vi "Receiver UI.vi"(8 "Error In":errorcluster) -> (0 "Error Out":errorcluster, 11 "Notification":bool)   [LabVIEW 2023, in "Receiver.lvclass"]
doc: "The VI receives data from sender and displays the received message of different data types."
uses:
  Receiver.lvclass
  Controls/Queue Operation.ctl
  Controls/User Event Operations.ctl
  Controls/Receiver Data.ctl
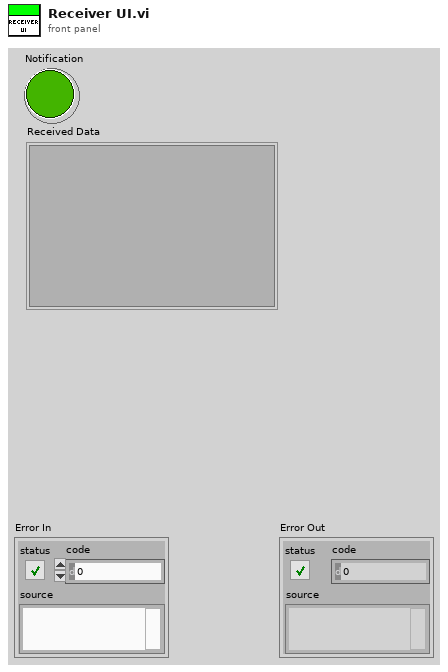
[diagram p1: front panel]
types:
  T1 = typedef "Receiver Data.ctl" = cluster{"Notification":bool, "Display Ref":refnum<vi>}
  T2 = typedef "User Event Operations.ctl" = enum16{"Obtain", "Generate", "Destroy"}
  T3 = typedef "Queue Operation.ctl" = enum16{"Create & Enqueue N", "Enqueue N", "Dequeue", "Enstack N", "Flush", "Release"}
  T4 = typedef "Queue Element.ctl" = cluster{"State":string, "Data":variant}
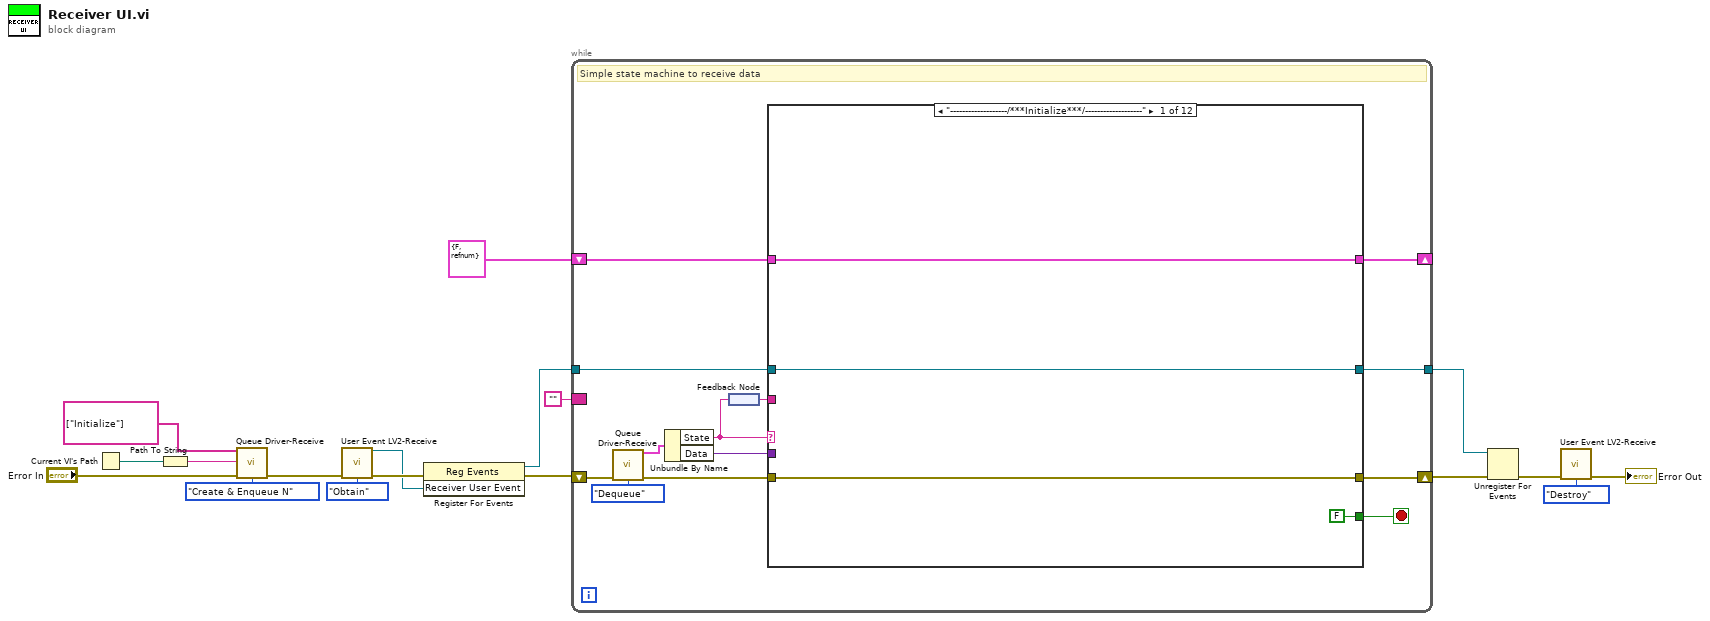
[diagram p0: block diagram]
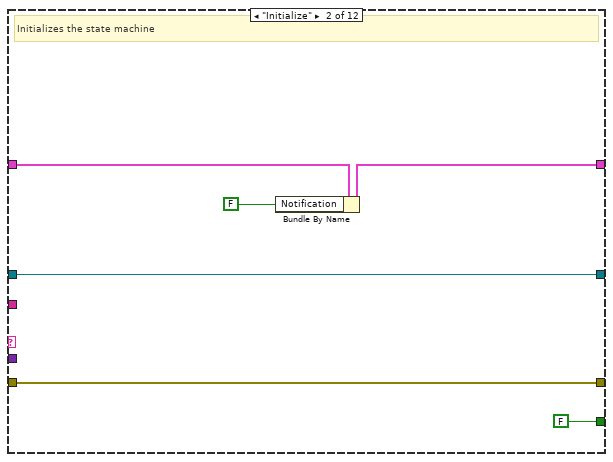
[diagram p2: hidden frame]
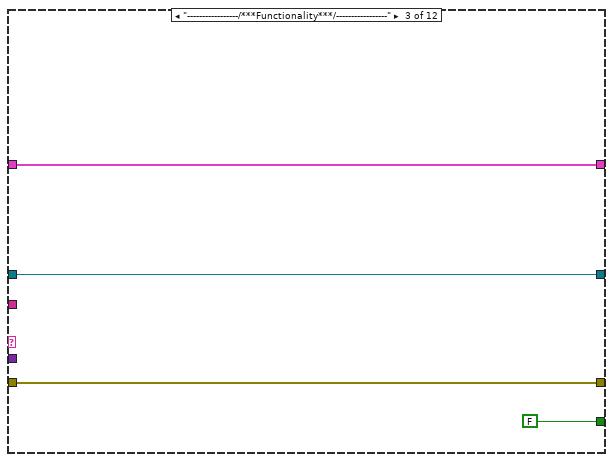
[diagram p3: hidden frame]
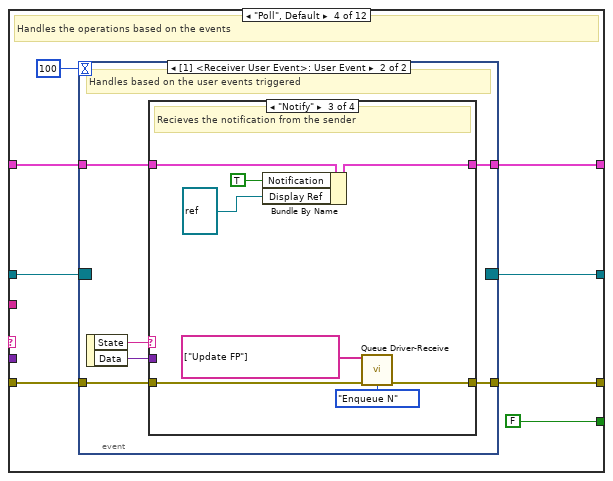
[diagram p4: hidden frame]
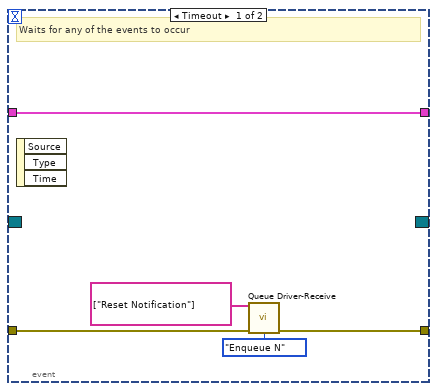
[diagram p5: hidden frame]
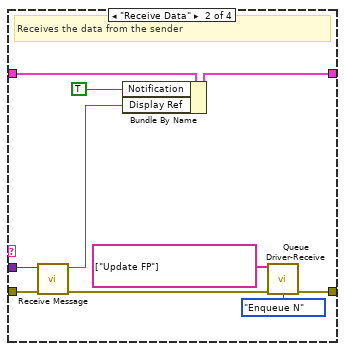
[diagram p7: hidden frame]
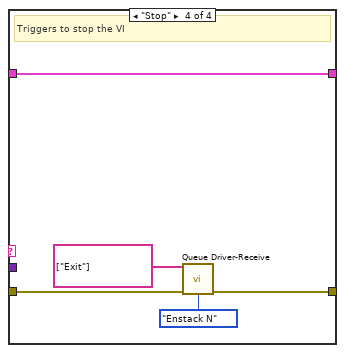
[diagram p8: hidden frame]
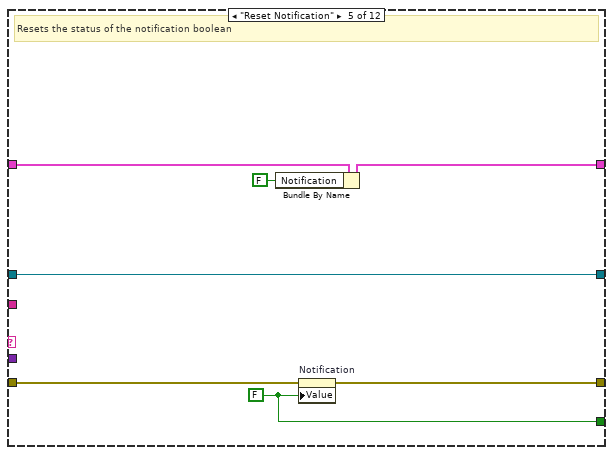
[diagram p9: hidden frame]
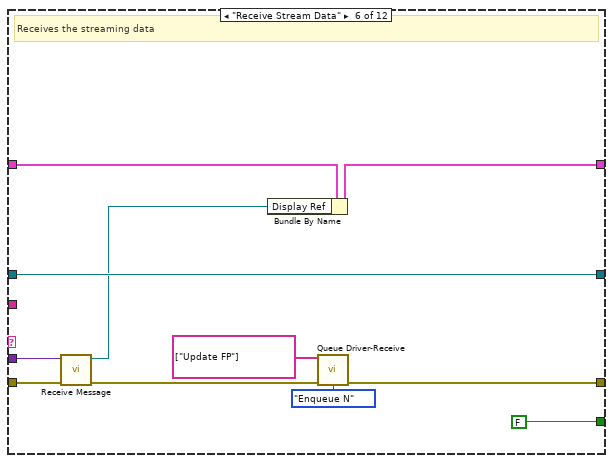
[diagram p10: hidden frame]
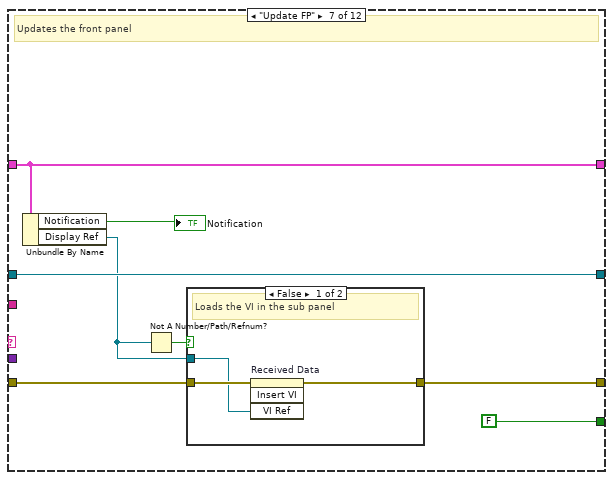
[diagram p11: hidden frame]
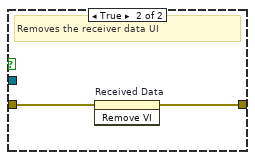
[diagram p12: hidden frame]
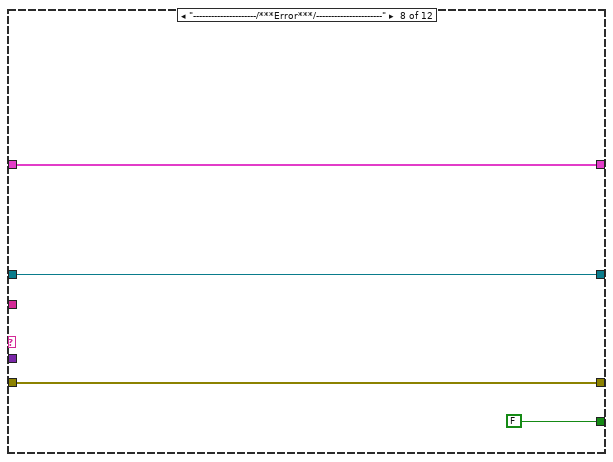
[diagram p13: hidden frame]
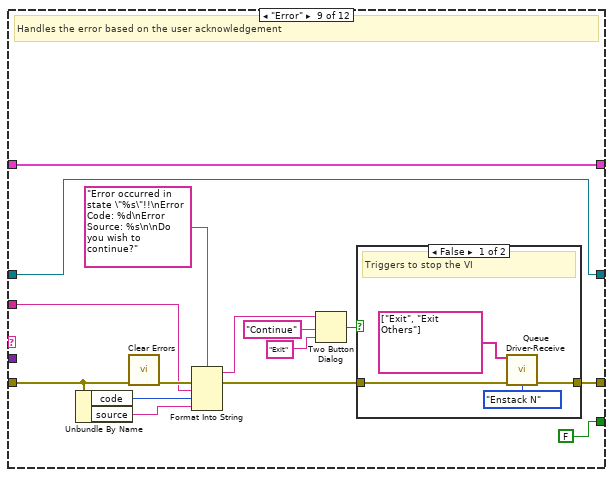
[diagram p14: hidden frame]
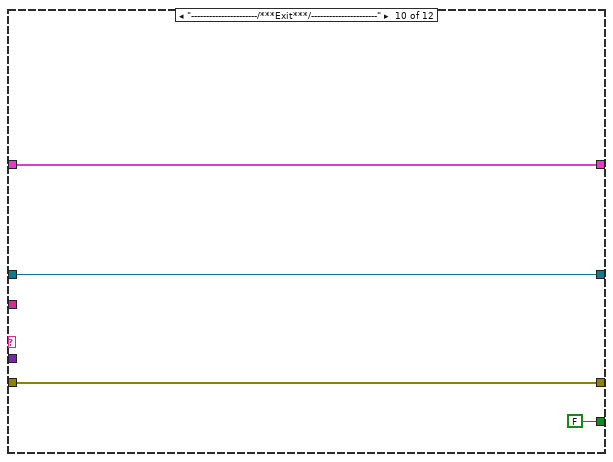
[diagram p16: hidden frame]
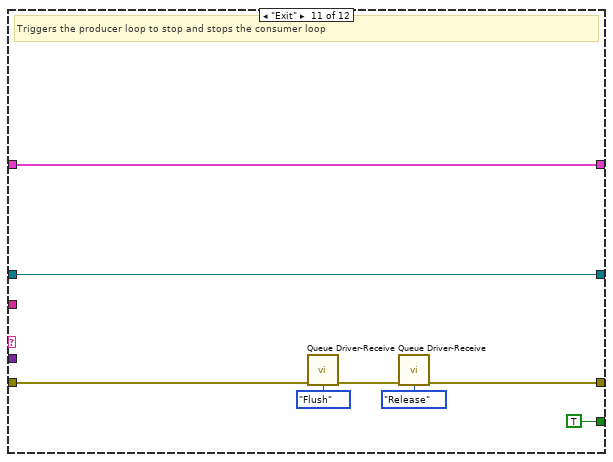
[diagram p17: hidden frame]
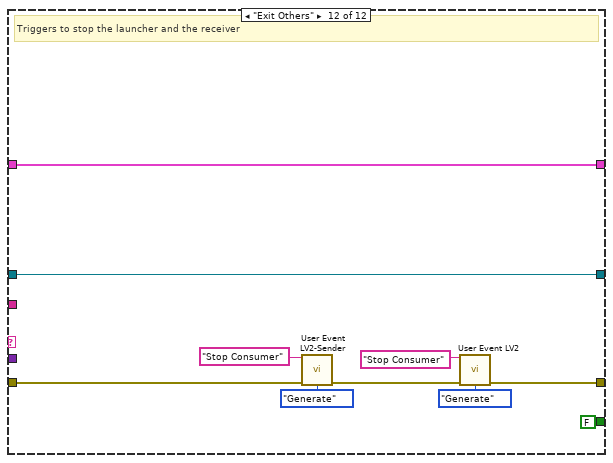
[diagram p18: hidden frame]
diagram:
  n1 = Current VI's Path() -> (path=w3:path)
  n2 = Path To String(path=w3) -> (string=w2:string)
  n3 = call "Queue Driver-Receive.vi"("States[]"=string[] ["Initialize"], "Queue Name"=w2, "Error In"="Error In", "Queue Operation"=Queue_Operation."Create & Enqueue N") -> ("Error Out"=w15:errorcluster)  [unwired: 10 in, 1 out]
  n4 = call "User Event LV2-Receive.vi"("Error In"=w15, "Operation"=User_Event_Operations."Obtain") -> ("Receiver User Event"=w9:refnum<user-event>, "Error Out"=w12:errorcluster)  [unwired: 12 in]
  n5 = register-events(error in=w12, w9) -> (reference out=w8:refnum<event-registration>, error out=w10:errorcluster)  [unwired: 1 in]
  n6 = while {
    shift-right: [w30] -> w16
    shift-left: w10 -> [w31]
    border: "" -> [_]
    tunnel: w8 -> [w23]
    tunnel: [w22] -> w6
    shift-right: [w19] -> _
    shift-left: T1 {"Notification"=FALSE, "Display Ref"=refnum} ("Receiver Data") -> [w20]
    stop <- w27 stop-if-true
    # "Simple state machine to receive data"
    n7 = call "Queue Driver-Receive.vi"("Error In"=w31, "Queue Operation"=Queue_Operation."Dequeue") -> ("Dequeue Element"=w21:T4, "Error Out"=w29:errorcluster)  [unwired: 12 in]
    n8 = Unbundle By Name(w21) -> ("State"=w26:string, "Data"=w24:variant)
    n9 = feedback-in #1(w26) -> ()
    n10 = feedback #1() -> (w25:string)
    n11 = case shown="\"-------------------/***Initialize***/-------------------\"" w26 {
      tunnel: w29 -> [w35 w36 w45 w53 w96 w102 w113 w124 w131 w148 w156 w166]
      tunnel: [w35 w36 w45 w51 w94 w105 w112 w124 w128 w148 w152 w161] -> w30
      tunnel: [FALSE FALSE FALSE FALSE w93 FALSE FALSE FALSE FALSE FALSE TRUE FALSE ("Notification")] -> w27
      tunnel: w25 -> [_ _ _ _ _ _ _ _ w129 _ _ _]
      tunnel: w24 -> [_ _ _ _ _ w100 _ _ _ _ _ _]
      tunnel: w23 -> [w33 w40 w43 w49 w95 w106 w114 w122 w126 w146 w150 w165]
      tunnel: [w33 w40 w43 w48 w95 w106 w114 w122 w126 w146 w150 w165] -> w22
      tunnel: w20 -> [w32 w39 w42 w47 w92 w99 w110 w121 w125 w145 w149 w157]
      tunnel: [w32 w38 w42 w46 w91 w98 w110 w121 w125 w145 w149 w157] -> w19
      frame "-------------------/***Initialize***/-------------------" {
      }
      frame "Initialize" {
        # "Initializes the state machine"
        n12 = Bundle By Name(cluster=w39, "Notification"=FALSE) -> (w38:T1)
      }
      frame "-----------------/***Functionality***/-----------------" {
      }
      frame "Poll", Default {
        # "Handles the operations based on the events"
        n13 = event shown="[1] <Receiver User Event>: User Event" {
          selector: w49 -> [_ _]
          dyn-events: [_ _] -> w48
          timeout: 100 -> [_ _]
          tunnel: w53 -> [w58 w64]
          tunnel: [w57 w63] -> w51
          tunnel: w47 -> [w54 w60]
          tunnel: [w54 w59] -> w46
          event Timeout {
            # "Waits for any of the events to occur"
            n14 = event-data() -> ()  [unwired: 1 in, 3 out]
            n15 = call "Queue Driver-Receive.vi"("States[]"=string[] ["Reset Notification"], "Error In"=w58, "Queue Operation"=Queue_Operation."Enqueue N") -> ("Error Out"=w57:errorcluster)  [unwired: 11 in, 1 out]
          }
          event User Event {
            # "Handles based on the user events triggered"
            n16 = event-data() -> ("State"=w62:string, "Data"=w61:variant)  [unwired: 1 in]
            n17 = case shown="\"Notify\"" w62 {
              tunnel: w64 -> [w66 w76 w84 w89]
              tunnel: [w66 w73 w83 w88] -> w63
              tunnel: w61 -> [_ w74 _ _]
              tunnel: w60 -> [w65 w70 w80 w85]
              tunnel: [w65 w69 w79 w85] -> w59
              frame Default {
                # "Do nothing"
              }
              frame "Receive Data" {
                # "Receives the data from the sender"
                n18 = call "Receive Message.vi"("Error In"=w76, "Data"=w74) -> ("Error Out"=w75:errorcluster, "Display Ref"=w67:refnum<vi>)  [unwired: 8 in]
                n19 = Bundle By Name(cluster=w70, "Notification"=TRUE, "Display Ref"=w67) -> (w69:T1)
                n20 = call "Queue Driver-Receive.vi"("States[]"=string[] ["Update FP"], "Error In"=w75, "Queue Operation"=Queue_Operation."Enqueue N") -> ("Error Out"=w73:errorcluster)  [unwired: 11 in, 1 out]
              }
              frame "Notify" {
                # "Recieves the notification from the sender"
                n21 = Bundle By Name(cluster=w80, "Notification"=TRUE, "Display Ref"=refnum<vi> refnum) -> (w79:T1)
                n22 = call "Queue Driver-Receive.vi"("States[]"=string[] ["Update FP"], "Error In"=w84, "Queue Operation"=Queue_Operation."Enqueue N") -> ("Error Out"=w83:errorcluster)  [unwired: 11 in, 1 out]
              }
              frame "Stop" {
                # "Triggers to stop the VI"
                n23 = call "Queue Driver-Receive.vi"("States[]"=string[] ["Exit"], "Error In"=w89, "Queue Operation"=Queue_Operation."Enstack N") -> ("Error Out"=w88:errorcluster)  [unwired: 11 in, 1 out]
              }
            }
          }
        }
      }
      frame "Reset Notification" {
        w93 = FALSE ("Notification")
        # "Resets the status of the notification boolean"
        n24 = Bundle By Name(cluster=w92, "Notification"=FALSE) -> (w91:T1)
        n25 = property on="Notification" class="Bool (strict)"(error in=w96, "Value"=w93) -> (error out=w94:errorcluster)  [unwired: 1 in, 1 out]
      }
      frame "Receive Stream Data" {
        # "Receives the streaming data"
        n26 = call "Receive Message.vi"("Error In"=w102, "Data"=w100) -> ("Error Out"=w101:errorcluster, "Display Ref"=w97:refnum<vi>)  [unwired: 8 in]
        n27 = Bundle By Name(cluster=w99, "Display Ref"=w97) -> (w98:T1)
        n28 = call "Queue Driver-Receive.vi"("States[]"=string[] ["Update FP"], "Error In"=w101, "Queue Operation"=Queue_Operation."Enqueue N") -> ("Error Out"=w105:errorcluster)  [unwired: 11 in, 1 out]
      }
      frame "Update FP" {
        # "Updates the front panel"
        n29 = Unbundle By Name(w110) -> ("Notification"=→"Notification":bool, "Display Ref"=w108:refnum<vi>)
        n30 = Not A Number/Path/Refnum?(number/path/refnum=w108) -> (NaN/Path/Refnum?=w111:bool)
        n31 = case shown="False" w111 {
          tunnel: [w118 w119] -> w112
          tunnel: w113 -> [w117 w120]
          tunnel: w108 -> [w116 _]
          frame False {
            # "Loads the VI in the sub panel"
            n32 = invoke on="Received Data" class="SubPnl" method="Insert VI"(error in=w117, "VI Ref"=w116) -> (error out=w118:errorcluster)  [unwired: 2 in, 3 out]
          }
          frame True {
            # "Removes the receiver data UI"
            n33 = invoke on="Received Data" class="SubPnl" method="Remove VI"(error in=w120) -> (error out=w119:errorcluster)  [unwired: 2 in, 2 out]
          }
        }
      }
      frame "---------------------/***Error***/----------------------" {
      }
      frame "Error" {
        # "Handles the error based on the user acknowledgement"
        n34 = Unbundle By Name(w131) -> ("code"=w133:i32, "source"=w132:string)
        n35 = call <vilib>:"Clear Errors.vi"("error in (no error)"=w131) -> ("error out"=w138:errorcluster)  [unwired: 5 in, 1 out]
        n36 = Format Into String(format string="Error occurred in state \"%s\"!!\nError Code: %d\nError Source: %s\n\nDo you wish to continue?", error in=w138, w129, w133, w132) -> (resulting string=w136:string, error out=w130:errorcluster)  [unwired: 1 in]
        n37 = Two Button Dialog(message=w136, 1:"Exit" ("F button name (\"Cancel\")"), 2:"Continue" ("T button name (\"OK\")")) -> (T button?=w127:bool)
        n38 = case shown="False" w127 {
          tunnel: w130 -> [w143 w144]
          tunnel: [w142 w144] -> w128
          frame False {
            # "Triggers to stop the VI"
            n39 = call "Queue Driver-Receive.vi"("States[]"=string[] ["Exit", "Exit Others"], "Error In"=w143, "Queue Operation"=Queue_Operation."Enstack N") -> ("Error Out"=w142:errorcluster)  [unwired: 11 in, 1 out]
          }
          frame True {
          }
        }
      }
      frame "----------------------/***Exit***/----------------------" {
      }
      frame "Exit" {
        # "Triggers the producer loop to stop and stops the consumer loop"
        n40 = call "Queue Driver-Receive.vi"("Error In"=w156, "Queue Operation"=Queue_Operation."Flush") -> ("Error Out"=w154:errorcluster)  [unwired: 12 in, 1 out]
        n41 = call "Queue Driver-Receive.vi"("Error In"=w154, "Queue Operation"=Queue_Operation."Release") -> ("Error Out"=w152:errorcluster)  [unwired: 12 in, 1 out]
      }
      frame "Exit Others" {
        # "Triggers to stop the launcher and the receiver"
        n42 = call "User Event LV2-Sender.vi"("Event Name"="Stop Consumer", "Error In"=w166, "Operation"=User_Event_Operations."Generate") -> ("Error Out"=w163:errorcluster)  [unwired: 11 in, 1 out]
        n43 = call "User Event LV2.vi"("Event Name"="Stop Consumer", "Error In"=w163, "Operation"=User_Event_Operations."Generate") -> ("Error Out"=w161:errorcluster)  [unwired: 11 in, 1 out]
      }
    }
  }
  n44 = Unregister For Events(event registration refnum=w6, error in=w16) -> (error out=w7:errorcluster)
  n45 = call "User Event LV2-Receive.vi"("Error In"=w7, "Operation"=User_Event_Operations."Destroy") -> ("Error Out"=→"Error Out":errorcluster)  [unwired: 12 in, 1 out]
